vi "Filter Setting Dialog.vi"(11 "Filter in":T1(array[cluster]) {"End" format="%x"; "Start" format="%x"}) -> (2 "Cancel?":bool, 3 "Filter out":T1(array[cluster]) {"End" format="%x"; "Start" format="%x"})   [LabVIEW 2018, in "CAN FD.lvlib"]
uses:
  CAN FD.lvlib
panel:
  in  "Cancel":bool
  in  "OK":bool
  in  "Del":bool
  in  "Add":bool
  in  "End":u32 caption="结束ID：0x" max=2047 format="%x"
  in  "Start":u32 caption="起始ID：0x" max=2047 format="%x"
  in  "Mode":enum16{"标准帧组ID", "标准帧明确ID", "扩展帧组ID", "扩展帧明确ID"}(ring) caption="模式："
  in  "List":i32(listbox)=-1
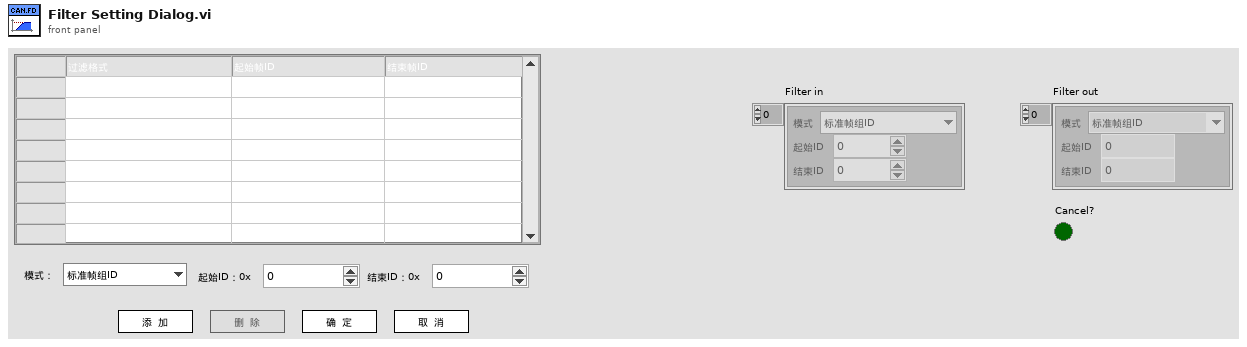
[diagram p1: front panel]
types:
  T1 = cluster{"Mode":enum16{"标准帧组ID", "标准帧明确ID", "扩展帧组ID", "扩展帧明确ID"}, "Start":u32, "End":u32}[]
  T2 = cluster{"Mode":enum16{"标准帧组ID", "标准帧明确ID", "扩展帧组ID", "扩展帧明确ID"}, "Start":u32, "End":u32}
  T3 = typedef "LVRowAndColumnUnsignedTypeDef.ctl" = cluster{"Row":u32, "Column":u32}
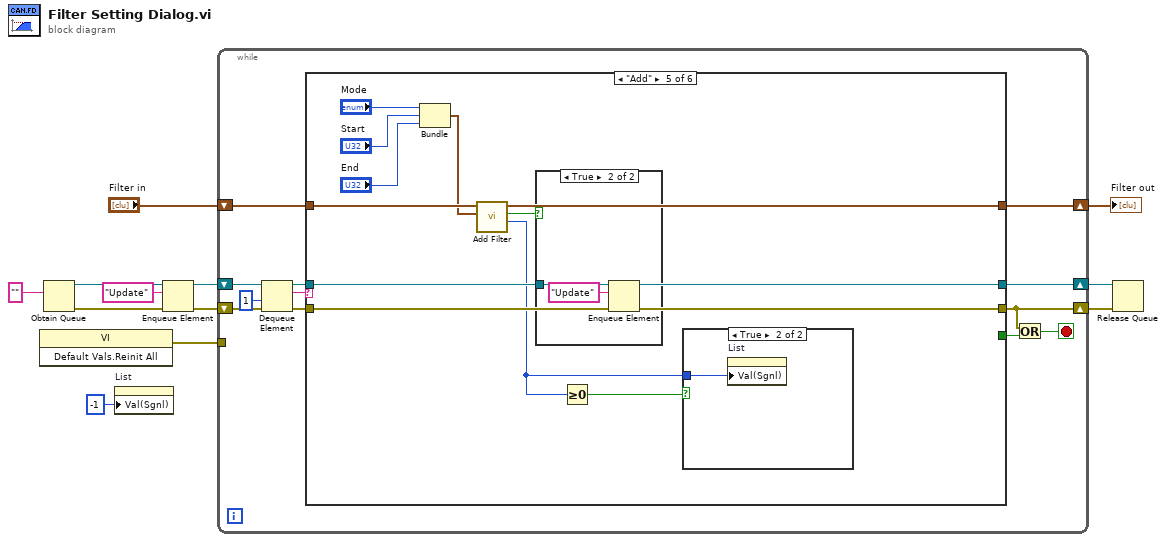
[diagram p0: block diagram]
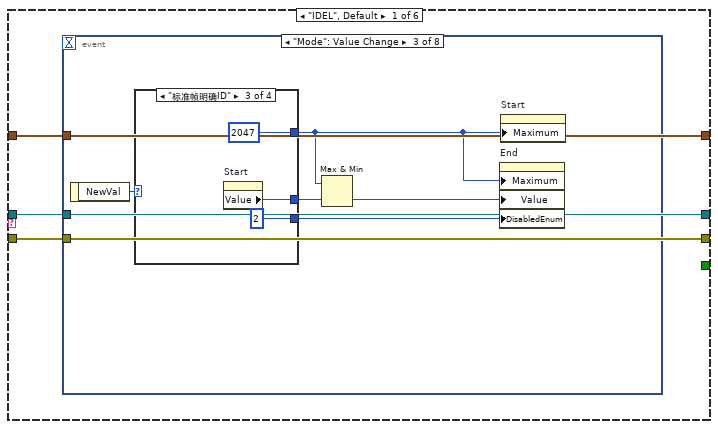
[diagram p2: hidden frame]
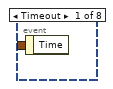
[diagram p3: hidden frame]
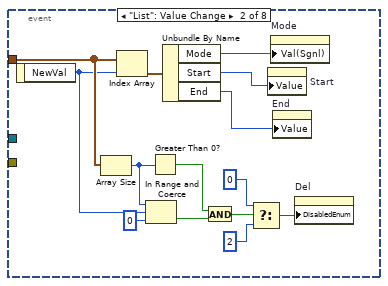
[diagram p4: hidden frame]
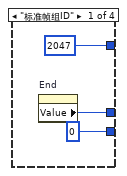
[diagram p5: hidden frame]
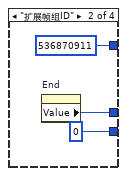
[diagram p6: hidden frame]
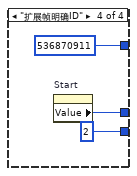
[diagram p7: hidden frame]
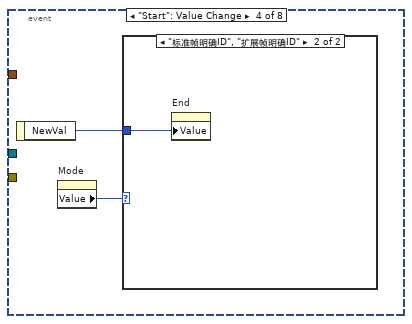
[diagram p8: hidden frame]
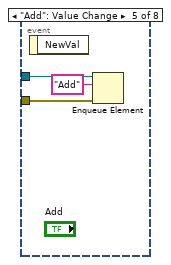
[diagram p10: hidden frame]
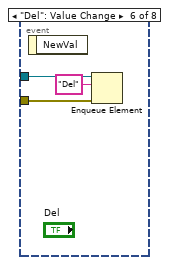
[diagram p11: hidden frame]
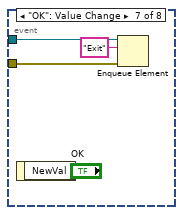
[diagram p12: hidden frame]
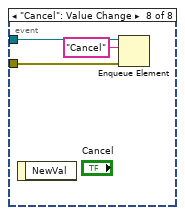
[diagram p13: hidden frame]
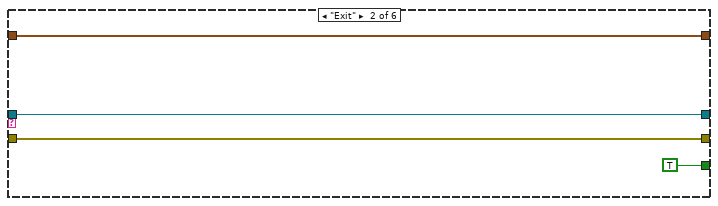
[diagram p14: hidden frame]
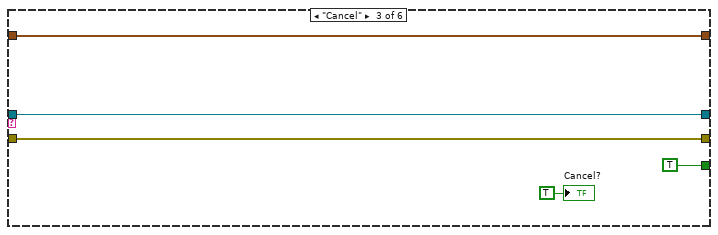
[diagram p15: hidden frame]
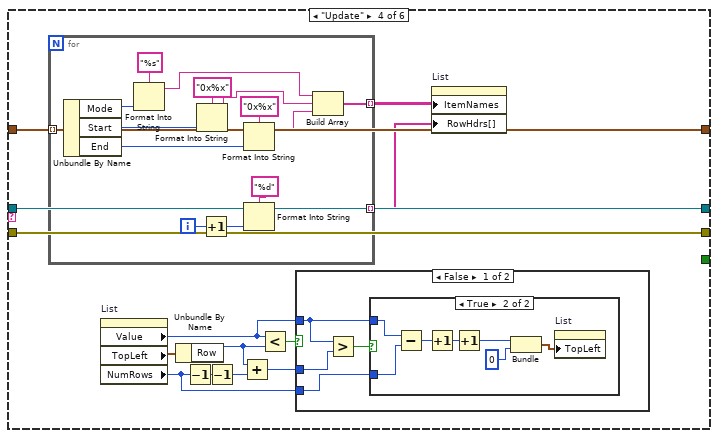
[diagram p16: hidden frame]
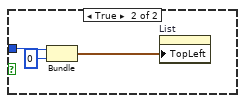
[diagram p18: hidden frame]
diagram:
  n1 = invoke class="VI" method="Default Vals.Reinit All"() -> (error out=w2:errorcluster)  [unwired: 3 in, 2 out]
  n2 = Obtain Queue(element data type="") -> (queue out=w9:refnum<queue>, error out=w7:errorcluster)  [unwired: 4 in, 1 out]
  n3 = property on="List" class="MCListbox (strict)"("Val(Sgnl)"=-1 ("List")) -> ()  [unwired: 2 in, 2 out]
  n4 = Enqueue Element(queue=w9, element="Update" ("元素"), error in (no error)=w7) -> (queue out=w8:refnum<queue>, error out=w6:errorcluster)  [unwired: 1 in, 1 out]
  n5 = while {
    shift-right: [w16] -> w11
    shift-left: "Filter in" -> [w20]
    shift-right: [w17] -> w4
    shift-left: w8 -> [w24]
    shift-right: [w14] -> w3
    shift-left: w6 -> [w23]
    tunnel: w2 -> [_]
    stop <- w13 stop-if-true
    n6 = Dequeue Element(queue=w24, timeout in ms (-1)=1 ("超时毫秒(-1)"), error in (no error)=w23) -> (queue out=w18:refnum<queue>, element=w21:string, error out=w19:errorcluster)  [unwired: 1 out]
    n7 = case shown="\"Add\"" w21 {
      tunnel: w20 -> [w25 w77 w82 w93 w131 w141]
      tunnel: w19 -> [w26 w76 w81 w95 w135 w149]
      tunnel: [w26 w76 w81 w95 w135 w149] -> w14
      tunnel: w18 -> [w27 w75 w80 w94 w127 w139]
      tunnel: [w27 w75 w80 w94 w127 w139] -> w17
      tunnel: [w25 w77 w82 w93 w130 w142] -> w16
      tunnel: [_ TRUE TRUE _ _ _] -> w15
      frame "IDEL", Default {
        n8 = event shown="[2] \"Mode\": Value Change" {
          selector: _ -> [_ _ _ _ _ _ _ _]
          dyn-events: _ -> [_ _ _ _ _ _ _ _]
          timeout: _ -> [_ _ _ _ _ _ _ _]
          tunnel: w27 -> [_ _ _ _ w64 w67 w70 w73]
          tunnel: w26 -> [_ _ _ _ w63 w66 w69 w72]
          tunnel: w25 -> [_ w37 _ _ _ _ _ _]
          event Timeout {
            n9 = event-data() -> ()  [unwired: 1 in, 1 out]
          }
          event "List": Value Change {
            n10 = event-data() -> ("NewVal"=w36:i32)  [unwired: 1 in]
            n11 = Array Size(array=w37) -> (size(s)=w34:i32)
            n12 = Index Array(array=w37, index=w36) -> (element=w41:T2)
            n13 = In Range and Coerce(upper limit=w34, x=w36, lower limit=0 ("下限")) -> (In Range?=w33:bool)  [unwired: 1 out]
            n14 = Greater Than 0?(x=w34) -> (x > 0?=w32:bool)
            n15 = Unbundle By Name(w41) -> ("Mode"=w40:enum16{"标准帧组ID", "标准帧明确ID", "扩展帧组ID", "扩展帧明确ID"}, "Start"=w39:u32, "End"=w38:u32)
            n16 = And(x=w32, y=w33) -> (x .and. y?=w31:bool)
            n17 = Select(t=0, s=w31, f=2) -> (s? t:f=w28:i32)
            n18 = property on="Start" class="DigNum (strict)"("Value"=w39) -> ()  [unwired: 2 in, 2 out]
            n19 = property on="Mode" class="Enum (strict)"("Val(Sgnl)"=w40) -> ()  [unwired: 2 in, 2 out]
            n20 = property on="End" class="DigNum (strict)"("Value"=w38) -> ()  [unwired: 2 in, 2 out]
            n21 = property on="Del" class="Bool"("DisabledEnum"=w28) -> ()  [unwired: 2 in, 2 out]
          }
          event "Mode": Value Change {
            n22 = event-data() -> ("NewVal"=w46:enum16{"标准帧组ID", "标准帧明确ID", "扩展帧组ID", "扩展帧明确ID"})  [unwired: 1 in]
            n23 = case shown="\"标准帧明确ID\"" w46 {
              tunnel: [u32 2047 ("Start") u32 536870911 ("Start") u32 2047 ("Start") u32 536870911 ("Start")] -> w43
              tunnel: [w48 w51 w54 w57] -> w44
              tunnel: [0 0 2 2] -> w45
              frame "标准帧组ID" {
                n24 = property on="End" class="DigNum (strict)"() -> ("Value"=w48:u32)  [unwired: 2 in, 2 out]
              }
              frame "扩展帧组ID" {
                n25 = property on="End" class="DigNum (strict)"() -> ("Value"=w51:u32)  [unwired: 2 in, 2 out]
              }
              frame "标准帧明确ID" {
                n26 = property on="Start" class="DigNum (strict)"() -> ("Value"=w54:u32)  [unwired: 2 in, 2 out]
              }
              frame "扩展帧明确ID" {
                n27 = property on="Start" class="DigNum (strict)"() -> ("Value"=w57:u32)  [unwired: 2 in, 2 out]
              }
            }
            n28 = Max & Min(x=w43, y=w44) -> (min(x,y)=w42:u32)  [unwired: 1 out]
            n29 = property on="End" class="DigNum (strict)"("Maximum"=w43, "Value"=w42, "DisabledEnum"=w45) -> ()  [unwired: 2 in, 2 out]
            n30 = property on="Start" class="DigNum (strict)"("Maximum"=w43) -> ()  [unwired: 2 in, 2 out]
          }
          event "Start": Value Change {
            n31 = event-data() -> ("NewVal"=w59:u32)  [unwired: 1 in]
            n32 = property on="Mode" class="Enum (strict)"() -> ("Value"=w60:enum16{"标准帧组ID", "标准帧明确ID", "扩展帧组ID", "扩展帧明确ID"})  [unwired: 2 in, 2 out]
            n33 = case shown="\"标准帧明确ID\", \"扩展帧明确ID\"" w60 {
              tunnel: w59 -> [_ w61]
              frame "标准帧组ID", Default {
              }
              frame "标准帧明确ID", "扩展帧明确ID" {
                n34 = property on="End" class="DigNum (strict)"("Value"=w61) -> ()  [unwired: 2 in, 2 out]
              }
            }
          }
          event "Add": Value Change {
            n35 = event-data() -> ()  [unwired: 1 in, 1 out]
            n36 = Enqueue Element(queue=w64, element="Add" ("元素"), error in (no error)=w63) -> ()  [unwired: 1 in, 3 out]
          }
          event "Del": Value Change {
            n37 = event-data() -> ()  [unwired: 1 in, 1 out]
            n38 = Enqueue Element(queue=w67, element="Del" ("元素"), error in (no error)=w66) -> ()  [unwired: 1 in, 3 out]
          }
          event "OK": Value Change {
            n39 = event-data() -> ()  [unwired: 1 in, 1 out]
            n40 = Enqueue Element(queue=w70, element="Exit" ("元素"), error in (no error)=w69) -> ()  [unwired: 1 in, 3 out]
          }
          event "Cancel": Value Change {
            n41 = event-data() -> ()  [unwired: 1 in, 1 out]
            n42 = Enqueue Element(queue=w73, element="Cancel" ("元素"), error in (no error)=w72) -> ()  [unwired: 1 in, 3 out]
          }
        }
      }
      frame "Exit" {
      }
      frame "Cancel" {
        "Cancel?" <- TRUE ("Cancel?")
      }
      frame "Update" {
        n43 = for {
          tunnel: w93 -> [w124] mode=indexing
          tunnel: [w114] -> w92 mode=indexing
          tunnel: [w110] -> w91 mode=indexing
          i -> [w112]
          n44 = Unbundle By Name(w124) -> ("Mode"=w123:enum16{"标准帧组ID", "标准帧明确ID", "扩展帧组ID", "扩展帧明确ID"}, "Start"=w121:u32, "End"=w118:u32)
          n45 = Format Into String(format string="%s" ("格式字符串"), w123) -> (resulting string=w117:string)  [unwired: 2 in, 1 out]
          n46 = Format Into String(format string="0x%x" ("格式字符串"), w121) -> (resulting string=w116:string)  [unwired: 2 in, 1 out]
          n47 = Increment(x=w112) -> (x+1=w111:i32)
          n48 = Format Into String(format string="0x%x" ("格式字符串"), w118) -> (resulting string=w115:string)  [unwired: 2 in, 1 out]
          n49 = Format Into String(format string="%d" ("格式字符串"), w111) -> (resulting string=w110:string)  [unwired: 2 in, 1 out]
          n50 = Build Array(w117, w116, w115) -> (w114:string[])
        }
        n51 = property on="List" class="MCListbox (strict)"() -> ("Value"=w88:i32, "TopLeft"=w90:T3, "NumRows"=w84:u32)  [unwired: 2 in, 2 out]
        n52 = Unbundle By Name(w90) -> ("Row"=w87:u32)
        n53 = Decrement(x=w84) -> (x-1=w85:u32)
        n54 = Decrement(x=w85) -> (x-1=w83:u32)
        n55 = Add(x=w87, y=w83) -> (x+y=w86:u32)
        n56 = Less?(x=w88, y=w87) -> (x < y?=w89:bool)
        n57 = case shown="False" w89 {
          tunnel: w88 -> [w97 w109]
          tunnel: w86 -> [w99 _]
          tunnel: w84 -> [w96 _]
          frame False {
            n58 = Greater?(x=w97, y=w99) -> (0:w98:bool)
            n59 = case shown="True" w98 {
              tunnel: w97 -> [_ w106]
              tunnel: w96 -> [_ w105]
              frame False {
              }
              frame True {
                n60 = Subtract(x=w106, y=w105) -> (x-y=w104:u32)
                n61 = Increment(x=w104) -> (x+1=w101:u32)
                n62 = Increment(x=w101) -> (x+1=w100:u32)
                n63 = Bundle(w100, 0) -> (w102:cluster{u32, i32})  [unwired: 1 in]
                n64 = property on="List" class="MCListbox (strict)"("TopLeft"=w102) -> ()  [unwired: 2 in, 2 out]
              }
            }
          }
          frame True {
            n65 = Bundle("Value"=w109, 0) -> (w107:cluster{"Value":i32, i32})  [unwired: 1 in]
            n66 = property on="List" class="MCListbox (strict)"("TopLeft"=w107) -> ()  [unwired: 2 in, 2 out]
          }
        }
        n67 = property on="List" class="MCListbox (strict)"("ItemNames"=w92, "RowHdrs[]"=w91) -> ()  [unwired: 2 in, 2 out]
      }
      frame "Add" {
        n68 = Bundle("Mode"="Mode", "Start"="Start", "End"="End") -> (w129:T2)  [unwired: 1 in]
        n69 = call "Add Filter.vi"("Filter"=w129, "Filter in"=w131) -> ("NewIndex"=w125:i32, "Success"=w128:bool, "Filter out"=w130:T1)  [unwired: 7 in]
        n70 = case shown="True" w128 {
          tunnel: w127 -> [_ w137]
          frame False {
          }
          frame True {
            n71 = Enqueue Element(queue=w137, element="Update" ("元素")) -> ()  [unwired: 2 in, 3 out]
          }
        }
        n72 = Greater Or Equal To 0?(x=w125) -> (x >= 0?=w126:bool)
        n73 = case shown="True" w126 {
          tunnel: w125 -> [_ w136]
          frame False {
          }
          frame True {
            n74 = property on="List" class="MCListbox (strict)"("Val(Sgnl)"=w136) -> ()  [unwired: 2 in, 2 out]
          }
        }
      }
      frame "Del" {
        n75 = Array Size(array=w141) -> (size(s)=w146:i32)
        n76 = In Range and Coerce(upper limit=w146, x="List", lower limit=0 ("下限")) -> (coerced(x)=w140:i32, In Range?=w145:bool)
        n77 = Greater Than 0?(x=w146) -> (x > 0?=w144:bool)
        n78 = And(x=w144, y=w145) -> (x .and. y?=w143:bool)
        n79 = case shown="True" w143 {
          tunnel: [w150 w153] -> w142
          tunnel: w141 -> [w150 w154]
          tunnel: w140 -> [_ w152]
          tunnel: w139 -> [_ w151]
          frame False {
          }
          frame True {
            n80 = Two Button Dialog(message="确定删除选中项？" ("消息")) -> (T button?=w155:bool)  [unwired: 2 in]
            n81 = case shown="True" w155 {
              tunnel: w154 -> [w157 w166]
              tunnel: [w157 w164] -> w153
              tunnel: w152 -> [_ w165]
              tunnel: w151 -> [_ w158]
              frame False {
              }
              frame True {
                n82 = Delete From Array(array=w166, index=w165) -> (array with subset deleted=w164:T1)  [unwired: 1 in, 1 out]
                n83 = Array Size(array=w164) -> (size(s)=w163:i32)
                n84 = Decrement(x=w163) -> (x-1=w162:i32)
                n85 = In Range and Coerce(upper limit=w162, x=w165, lower limit=0 ("下限")) -> (coerced(x)=w160:i32)  [unwired: 1 out]
                n86 = Enqueue Element(queue=w158, element="Update" ("元素")) -> ()  [unwired: 2 in, 3 out]
                n87 = property on="List" class="MCListbox (strict)"("Val(Sgnl)"=w160) -> ()  [unwired: 2 in, 2 out]
              }
            }
          }
        }
      }
    }
    n88 = Or(x=w14, y=w15) -> (x .or. y?=w13:bool)
  }
  "Filter out" <- w11
  n89 = Release Queue(queue=w4, error in (no error)=w3) -> ()  [unwired: 1 in, 3 out]
